vi "Set Bitmap.vi"(8 "error in (no error)":errorcluster, 10 "Bitmap":u32[][](array[numeric]), 11 "Listbox Icon Canvas in":refnum<class "Listbox Icon Canvas.lvclass">) -> (0 "error out":errorcluster, 3 "Listbox Icon Canvas out":refnum<class "Listbox Icon Canvas.lvclass">)   [LabVIEW 2020, in "Glyph Drawer.lvlib" / "Listbox Icon Canvas.lvclass"]
uses:
  Listbox Icon Canvas.lvclass
  Listbox Icon Canvas.lvclass/Listbox Icon Canvas.ctl
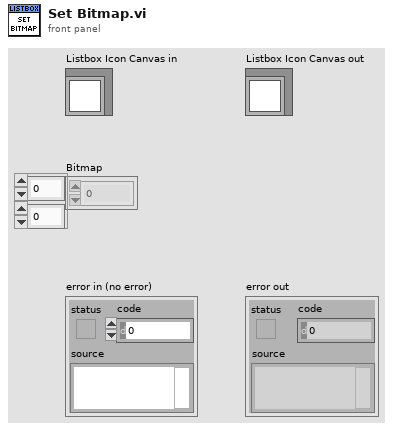
[diagram p1: front panel]
types:
  T1 = typedef "imagedata.ctl" = cluster{"image type":i32, "image depth":i32, "image":u8[], "mask":u8[], "colors":u32[], "Rectangle":cluster{"left":i16, "top":i16, "right":i16, "bottom":i16}}
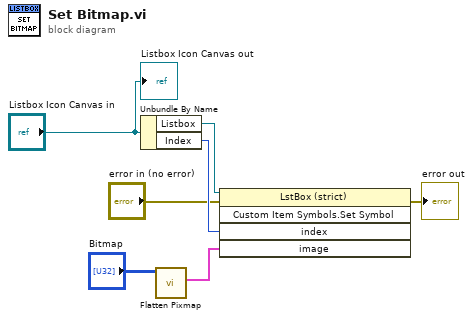
[diagram p0: block diagram]
diagram:
  n1 = Unbundle By Name("Listbox Icon Canvas in") -> ("Listbox"=w6:refnum<vi>, "Index"=w5:i32)
  n2 = call <vilib>:"Flatten Pixmap.vi"("24-bit pixmap"="Bitmap") -> ("image data"=w3:T1)  [unwired: 10 in]
  n3 = invoke class="LstBox (strict)" method="Custom Item Symbols.Set Symbol"(reference=w6, error in="error in (no error)", "index"=w5, "image"=w3) -> (error out=→"error out":errorcluster)  [unwired: 1 in, 4 out]
  "Listbox Icon Canvas out" <- "Listbox Icon Canvas in"
